vi "MGCC_MdlMgmt_converttopology.vi"() -> ()   [LabVIEW 2016]
doc: "-----------------------------------------------------------------------------------------------------------------------\nCopyright <2019> <The University of Tennessee at Knoxville and the University of Tennessee Research Foundation>\nThis software is released under BSD-3 \nhttps://opensource.org/licenses/BSD-3-Clause \nAdditional license options available at https://utrf.tennessee.edu/industry/sample-agreements/\n-----------------------------------------------------------------------------------------------------------------------"
uses:
  Global_MdlMgmt.vi
  <vilib>/imath/engines/lvmath2/RunTimeEngine/IndexRead/NIMS M($,S).vi
  <instcachedir>/0/NIMS M($,S)_3E5749BBB62E49528D4765A77F1F6D98.lvgen/NIMS M($,S)_3E5749BBB62E49528D4765A77F1F6D98_000.vi
  <vilib>/imath/engines/lvmath2/RunTimeEngine/BuiltInFunctions/max/1 input/NIMS_max(RV).vi
  <instcachedir>/0/NIMS_max(RV)_237633DB1D604D5BA7001287DF3C7957.lvgen/NIMS_max(RV)_237633DB1D604D5BA7001287DF3C7957_000.vi
  <vilib>/imath/engines/lvmath2/RunTimeEngine/BuiltInFunctions/max/2 inputs/NIMS_max(RG,RG)-no size check.vi
  <instcachedir>/0/NIMS_max(RG,RG)-no size check_F871939977644B7683C1350DCCAD7557.lvgen/NIMS_max(RG,RG)-no size check_F871939977644B7683C1350DCCAD7557_000.vi
  <vilib>/imath/engines/lvmath2/RunTimeEngine/ErrorHandling/NIMS_Create Error From Enums.vi
  <vilib>/imath/engines/lvmath2/RunTimeEngine/BuiltInFunctions/length/NIMS_length(GM).vi
  <instcachedir>/0/NIMS_length(GM)_47CEC356FCE0482D9BA47DC61C99F2C7.lvgen/NIMS_length(GM)_47CEC356FCE0482D9BA47DC61C99F2C7_000.vi
  <vilib>/imath/engines/lvmath2/RunTimeEngine/MatrixToken/NIMS_MatrixToken_M_RV.vi
  <instcachedir>/0/NIMS_MatrixToken_M_RV_EE14907D4B194E829889005D2F556E9C.lvgen/NIMS_MatrixToken_M_RV_EE14907D4B194E829889005D2F556E9C_001.vi
  <vilib>/imathl/engines/lvmath/Functions/Error Handling/Create Error.vi
  <vilib>/imath/engines/lvmath2/RunTimeEngine/RangeToken/NIMS_Range_R3 - Integer.vi
  <instcachedir>/0/NIMS_Range_R3 - Integer_A435E2FF893B4C718FD5055FE39FE2F6.lvgen/NIMS_Range_R3 - Integer_A435E2FF893B4C718FD5055FE39FE2F6_000.vi
  <vilib>/imath/engines/lvmath2/RunTimeEngine/CommandStatement/MC_CommandStatement_break.vi
  <vilib>/imath/engines/lvmath2/RunTimeEngine/IndexRead/NIMS M(S,S).vi
  <instcachedir>/0/NIMS M(S,S)_AC51E74150A542F7991B9634C66F3096.lvgen/NIMS M(S,S)_AC51E74150A542F7991B9634C66F3096_000.vi
  <vilib>/imath/engines/lvmath2/RunTimeEngine/IndexReplace/NIMS M(S,S)=S.vi
  <instcachedir>/0/NIMS M(S,S)=S_98E40400474E4398B113AE20298B4F82.lvgen/NIMS M(S,S)=S_98E40400474E4398B113AE20298B4F82_000.vi
  <vilib>/imath/engines/lvmath2/RunTimeEngine/VariableToken/NIMS_VariableToken_CondDefinedDefinedByReplace.vi
  <instcachedir>/0/NIMS_VariableToken_CondDefinedDefinedByReplace_D162CFFC24174562A9FEA619A91E1A56.lvgen/NIMS_VariableToken_CondDefinedDefinedByReplace_D162CFFC24174562A9FEA619A91E1A56_001.vi
  <vilib>/imath/engines/lvmath2/RunTimeEngine/IndexRead/NIMS M(S,$).vi
  <instcachedir>/0/NIMS M(S,$)_F24F360562DE41D8BE234322A2E15C65.lvgen/NIMS M(S,$)_F24F360562DE41D8BE234322A2E15C65_000.vi
  <vilib>/imath/engines/lvmath2/RunTimeEngine/IndexReplace/NIMS M(S,$)=V.vi
  <instcachedir>/0/NIMS M(S,$)=V_BCCFA522A894489B8FA760383D74A164.lvgen/NIMS M(S,$)=V_BCCFA522A894489B8FA760383D74A164_000.vi
  <vilib>/imath/engines/lvmath2/RunTimeEngine/VariableToken/NIMS_VariableToken_CondDefined.vi
  <instcachedir>/0/NIMS_VariableToken_CondDefined_06E9DA95BD4D46A6BA55EC651A891960.lvgen/NIMS_VariableToken_CondDefined_06E9DA95BD4D46A6BA55EC651A891960_001.vi
  <vilib>/imath/engines/lvmath/Functions/Error Handling/MergeErrorsWrapper.vi
  <vilib>/imath/engines/lvmath2/RunTimeEngine/NodeEndStatement/NIMS_NodeEndStatement_Output.vi
  <instcachedir>/0/NIMS_NodeEndStatement_Output_53EC0D466D134D7ABD903AC30B43404B.lvgen/NIMS_NodeEndStatement_Output_53EC0D466D134D7ABD903AC30B43404B_002.vi
  <vilib>/imath/engines/lvmath2/RunTimeEngine/ErrorHandling/NIMS_Finalize Error.vi
  <vilib>/imath/engines/lvmath2/RunTimeEngine/Managers/WorkSpace/UID Generator.vi
  <vilib>/imath/engines/lvmath2/RunTimeEngine/BuiltInFunctions/size/NIMS_I32=size(GM,I32).vi
  <instcachedir>/0/NIMS_I32=size(GM,I32)_122058B1B3294FAEA5DC209B92B394E4.lvgen/NIMS_I32=size(GM,I32)_122058B1B3294FAEA5DC209B92B394E4_004.vi
  <vilib>/imath/engines/lvmath2/RunTimeEngine/RangeToken/NIMS_Range_R2 - Integer.vi
  <instcachedir>/0/NIMS_Range_R2 - Integer_89B873E74E6E489885E44F751DD9C6BF.lvgen/NIMS_Range_R2 - Integer_89B873E74E6E489885E44F751DD9C6BF_000.vi
  <vilib>/imath/engines/lvmath2/RunTimeEngine/IndexRead/NIMS V(S).vi
  <instcachedir>/0/NIMS V(S)_0488751826AF41519A22953C041130DC.lvgen/NIMS V(S)_0488751826AF41519A22953C041130DC_000.vi
  <vilib>/imath/engines/lvmath2/RunTimeEngine/IndexReplace/NIMS V(S)=S.vi
  <instcachedir>/0/NIMS V(S)=S_57E16554CB8B4B90AAB163894F717546.lvgen/NIMS V(S)=S_57E16554CB8B4B90AAB163894F717546_000.vi
  <vilib>/imath/engines/lvmath2/RunTimeEngine/RunTimeType/NIMS_RunTimeType_From StrictType (excl LVString).vi
  <instcachedir>/0/NIMS_RunTimeType_From StrictType (excl LVString)_BBF44FB49F834B71AF7A14CCEDF8BECD.lvgen/NIMS_RunTimeType_From StrictType (excl LVString)_BBF44FB49F834B71AF7A14CCEDF8BECD_000.vi
  <vilib>/imath/engines/lvmath2/RunTimeEngine/LocalVariableDefStatement/MC_LocalVariableDefStatement_Display.vi
  <vilib>/imath/engines/lvmath2/RunTimeEngine/Managers/SymbolTable/Clear UID.vi
  <instcachedir>/0/NIMS_NodeEndStatement_Output_53EC0D466D134D7ABD903AC30B43404B.lvgen/NIMS_NodeEndStatement_Output_53EC0D466D134D7ABD903AC30B43404B_005.vi
  <vilib>/imath/engines/lvmath2/RunTimeEngine/Managers/SymbolTable/NIMS_WorkSpace.lvlib
panel:
  out "error out":errorcluster
  in  "Topology":dbl[][](array[numeric])=[[2.0, 1.0, 3.0, 0.0, 100.0, 0.0, 0.0, 0.0, 0.0, 0.0, 0.0, 0.0, 0.0, 0.0, 0.0, 0.0], [3.0, 2.0, 1.0, 0.0, 1.0, 0.0, 0.0, 0.0, 0.0, 0.0, 0.0, 0.0, 0.0, 0.0, 0.0, 0.0], [3.0, 4.0, 1.0, 0.0, 2.0, 0.0, 0.0, 0.0, 0.0, 0.0, 0.0, 0.0, 0.0, 0.0, 0.0, 0.0], [4.0, 5.0, 1.0, 0.0, 4.0, 0.0, 0.0, 0.0, 0.0, 0.0, 0.0, 0.0, 0.0, 0.0, 0.0, 0.0], [4.0, 6.0, 3.0, 0.0, 100.0, 0.0, 0.0, 0.0, 0.0, 0.0, 0.0, 2.0, 1.0, 3.0, 0.0, 100.0], [7.0, 3.0, 1.0, 0.0, 3.0, 0.0, 0.0, 0.0, 0.0, 0.0, 0.0, 3.0, 2.0, 1.0, 0.0, 1.0], [7.0, 8.0, 1.0, 0.0, 5.0, 0.0, 0.0, 0.0, 0.0, 0.0, 0.0, 3.0, 4.0, 1.0, 0.0, 2.0], [9.0, 7.0, 1.0, 0.0, 6.0, 0.0, 0.0, 0.0, 0.0, 0.0, 0.0, 4.0, 5.0, 1.0, 0.0, 4.0], [10.0, 9.0, 1.0, 0.0, 7.0, 0.0, 0.0, 0.0, 0.0, 0.0, 0.0, 4.0, 6.0, 3.0, 0.0, 100.0], [10.0, 13.0, 3.0, 0.0, 100.0, 0.0, 0.0, 0.0, 0.0, 0.0, 0.0, 7.0, 3.0, 1.0, 0.0, 3.0], [10.0, 12.0, 3.0, 0.0, 100.0, 0.0, 0.0, 0.0, 0.0, 0.0, 0.0, 8.0, 7.0, 1.0, 0.0, 5.0], [10.0, 11.0, 1.0, 0.0, 8.0, 0.0, 0.0, 0.0, 0.0, 0.0, 0.0, 9.0, 7.0, 1.0, 0.0, 6.0], [11.0, 14.0, 3.0, 0.0, 100.0, 0.0, 0.0, 0.0, 0.0, 0.0, 0.0, 10.0, 9.0, 1.0, 0.0, 7.0], [0.0, 0.0, 0.0, 0.0, 0.0, 0.0, 0.0, 0.0, 0.0, 0.0, 0.0, 10.0, 13.0, 2.0, 0.0, 100.0], [0.0, 0.0, 0.0, 0.0, 0.0, 0.0, 0.0, 0.0, 0.0, 0.0, 0.0, 10.0, 12.0, 2.0, 0.0, 100.0], [0.0, 0.0, 0.0, 0.0, 0.0, 0.0, 0.0, 0.0, 0.0, 0.0, 0.0, 10.0, 11.0, 1.0, 0.0, 8.0], [0.0, 0.0, 0.0, 0.0, 0.0, 0.0, 0.0, 0.0, 0.0, 0.0, 0.0, 11.0, 14.0, 3.0, 0.0, 100.0]]
  out "Equal_M":dbl[][](array[numeric])
  out "Microgrid Topology Overall":dbl[][](array[numeric])
  out "array w/ subset deleted":dbl[][](array[numeric])
  out "Topology_identification":dbl[][](array[numeric])
  out "Topology_overall":dbl[][](array[numeric])
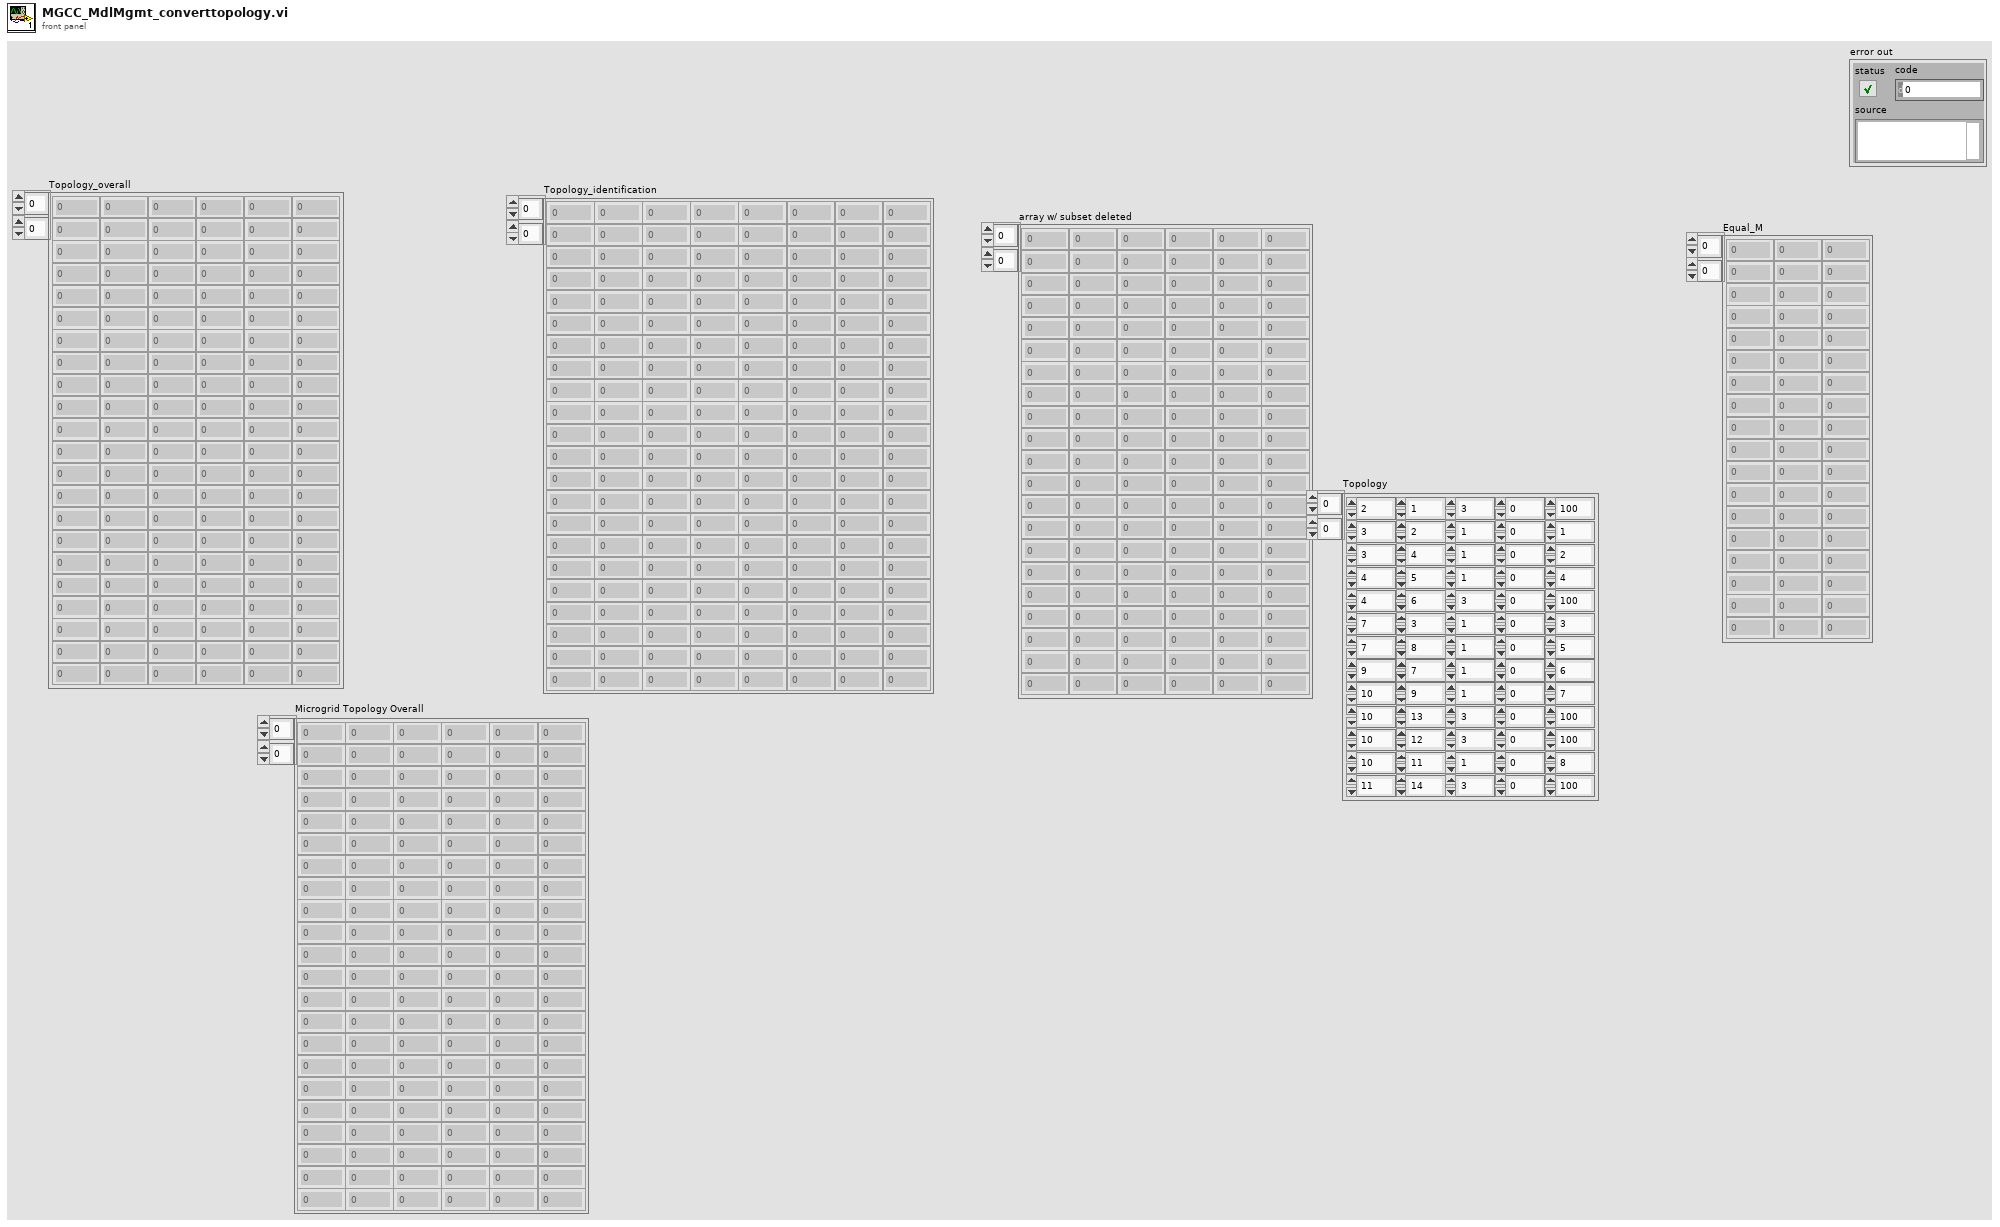
[diagram p1: front panel]
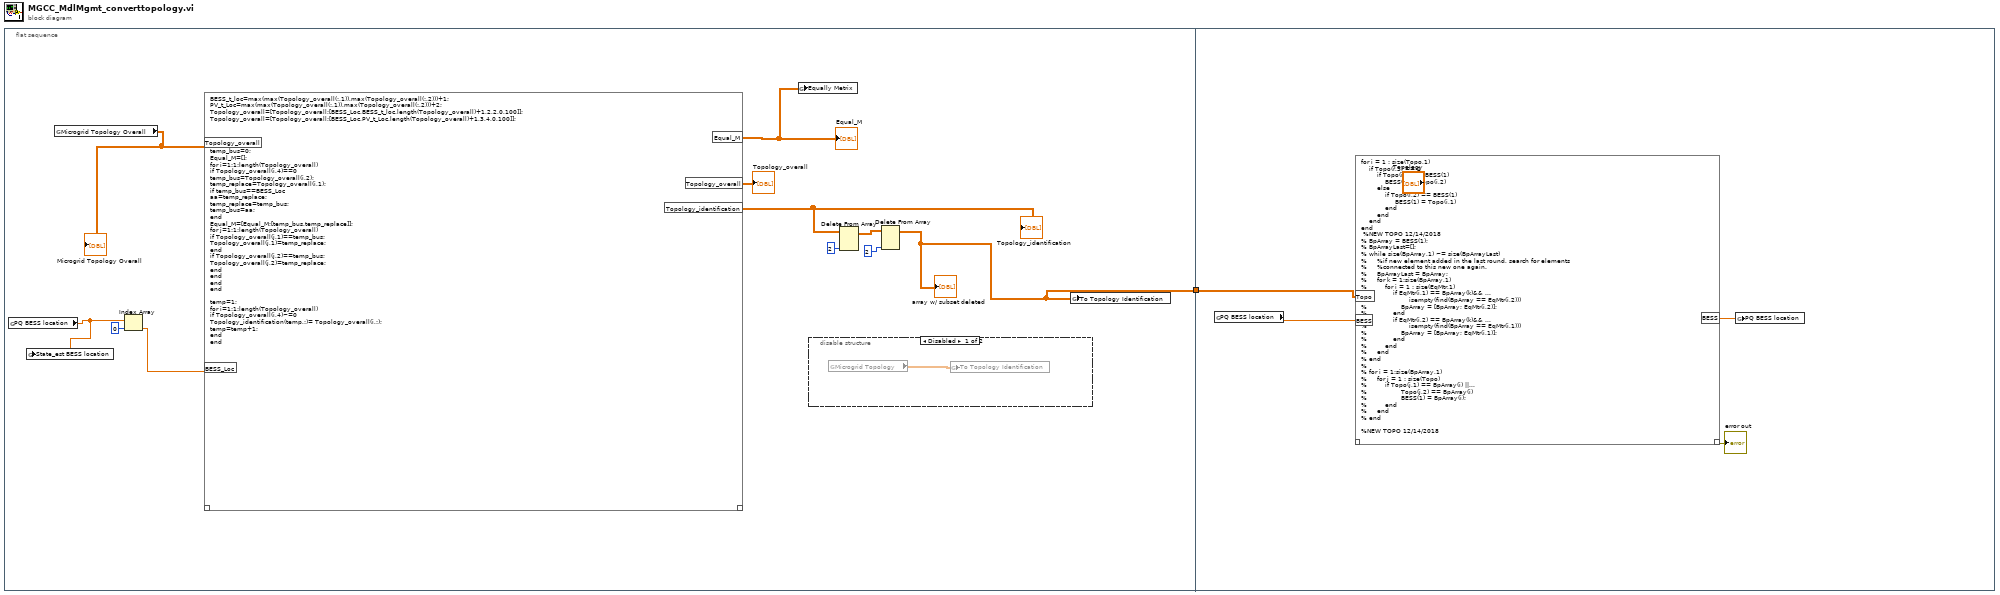
[diagram p0: block diagram]
diagram:
  n1 = flat-sequence {
    tunnel: [w2] -> w1
    tunnel: w1 -> [w658]
    frame #0 {
      n2 = global read "Global_MdlMgmt.vi" "PQ BESS location"() -> (w3:dbl[])
      n3 = global write "Global_MdlMgmt.vi" "State_est BESS location"(w3) -> ()
      n4 = global read "Global_MdlMgmt.vi" "Microgrid Topology Overall"() -> (w12:dbl[][])
      "Microgrid Topology Overall" <- w12
      n5 = Index Array(array=w3, index=0) -> (element=w4:dbl)
      n6 = mathscript code="BESS_t_loc=max(max(Topology_overall(:,1)),max(Topology_overall(:,2)))+1;\nPV_t_Loc=max(max(Topology_overall(:,1)),max(Topology_overall(:,2)))+2;\nTopology_overall=[Topology_overall;[BESS_Loc,BESS_t_loc,length(Topology_overall)+1,2,2,0,100]];\nTopology_overall=[Topology_overall;[BESS_Loc,PV_t_Loc,length(Topology_overall)+1,3,4,0,100]];\n\n\n\n\ntemp_bus=0;\nEqual_M=[];\nfor i=1:1:length(Topology_overall)\nif Topology_overall(i,4)==0\ntemp_bus=Topology_overall(i,2);\ntemp_replace=Topology_overall(i,1);\nif temp_bus==BESS_Loc\naa=temp_replace;\ntemp_replace=temp_bus;\ntemp_bus=aa;\nend\nEqual_M=[Equal_M;[temp_bus,temp_replace]];\nfor j=1:1:length(Topology_overall)\nif Topology_overall(j,1)==temp_bus;\nTopology_overall(j,1)=temp_replace;\nend\nif Topology_overall(j,2)==temp_bus;\nTopology_overall(j,2)=temp_replace;\nend\nend\nend\nend\n\ntemp=1;\nfor i=1:1:length(Topology_overall)\nif Topology_overall(i,4)~=0\nTopology_identification(temp,:)= Topology_overall(i,:);\ntemp=temp+1;\nend\nend"("Topology_overall"=w12, "BESS_Loc"=w4) -> ("Topology_overall"=→"Topology_overall":dbl[][], "Topology_identification"=w6:dbl[][], "Equal_M"=w7:dbl[][])  [unwired: 1 in, 1 out]
      "Topology_identification" <- w6
      "Equal_M" <- w7
      n7 = global write "Global_MdlMgmt.vi" "Equally Metrix"(w7) -> ()
      n8 = disable-structure shown="Disabled" {
        frame Disabled {
          n9 = global read "Global_MdlMgmt.vi" "Microgrid Topology"() -> (w13:dbl[][])
          n10 = global write "Global_MdlMgmt.vi" "To Topology Identification"(w13) -> ()
        }
        frame Enabled {
        }
      }
      n11 = Delete From Array(array=w6, index (col)=2 ("disabled index (col)")) -> (array with subset deleted=w9:dbl[][])  [unwired: 2 in, 1 out]
      n12 = Delete From Array(array=w9, index (col)=2 ("disabled index (col)")) -> (array with subset deleted=w2:dbl[][])  [unwired: 2 in, 1 out]
      "array w/ subset deleted" <- w2
      n13 = global write "Global_MdlMgmt.vi" "To Topology Identification"(w2) -> ()
    }
    frame #1 {
      n14 = global read "Global_MdlMgmt.vi" "PQ BESS location"() -> (w661:dbl[])
      n15 = mathscript code="for i = 1 : size(Topo,1)\n    if Topo(i,3) == 2\n        if Topo(i,1) == BESS(1)\n            BESS(1) = Topo(i,2)\n        else\n            if Topo(i,2) == BESS(1)\n                 BESS(1) = Topo(i,1)\n            end\n        end        \n    end\nend\n %NEW TOPO 12/14/2018\n% BpArray = BESS(1);\n% BpArrayLast=[];\n% while size(BpArray,1) ~= size(BpArrayLast)\n%     %if new element added in the last round, search for elements\n%     %connected to this new one again.\n%     BpArrayLast = BpArray;\n%     for k = 1:size(BpArray,1)\n%         for i = 1 : size(EqMtr,1)\n%             if EqMtr(i,1) == BpArray(k)&& ...\n%                     isempty(find(BpArray == EqMtr(i,2)))\n%                 BpArray = [BpArray; EqMtr(i,2)];\n%             end\n%             if EqMtr(i,2) == BpArray(k)&& ...\n%                     isempty(find(BpArray == EqMtr(i,1)))\n%                 BpArray = [BpArray; EqMtr(i,1)];\n%             end\n%         end\n%     end\n% end\n% \n% for i = 1:size(BpArray,1)\n%     for j = 1 : size(Topo)\n%         if Topo(j,1) == BpArray(i) ||...\n%                 Topo(j,2) == BpArray(i)\n%                 BESS(1) = BpArray(i);\n%         end\n%     end\n% end\n\n%NEW TOPO 12/14/2018"("Topo"=w658, "BESS"=w661) -> ("??"=→"error out":errorcluster, "BESS"=w659:dbl[])  [unwired: 1 in]
      n16 = global write "Global_MdlMgmt.vi" "PQ BESS location"(w659) -> ()
    }
  }
